vi "Update Count.vi"(8 "error in (no error)":errorcluster, 10 "Count":u64, 11 "Work Logic in":refnum<class "Work Logic.lvclass">) -> (0 "error out":errorcluster, 3 "Work Logic out":refnum<class "Work Logic.lvclass">)   [LabVIEW 2024, in "Chef State Logic.lvlib" / "Work Logic.lvclass"]
uses:
  Work Logic.lvclass
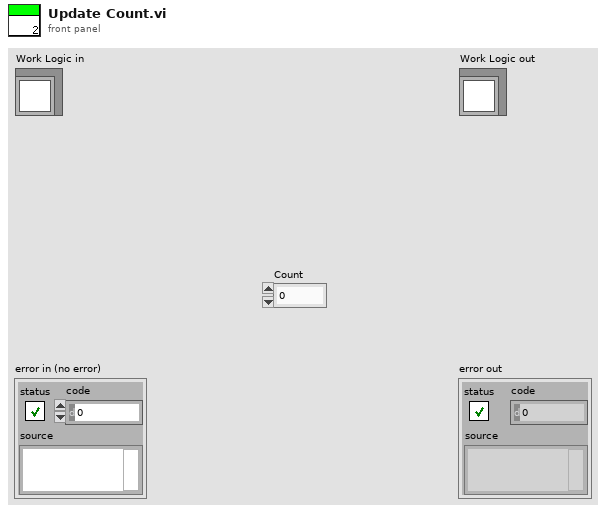
[diagram p1: front panel]
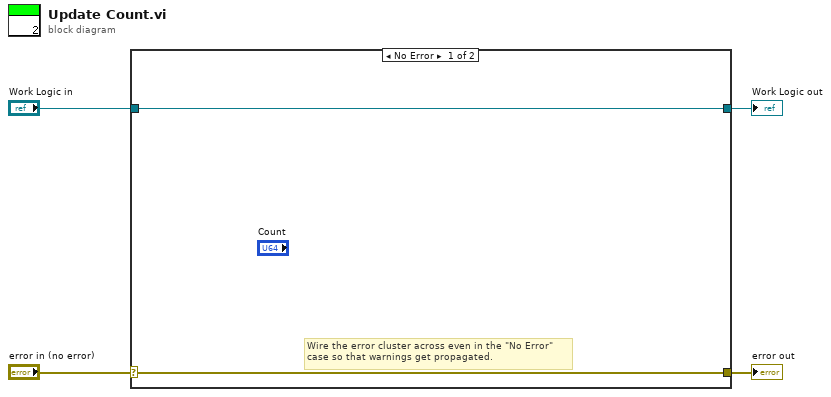
[diagram p0: block diagram]
diagram:
  n1 = case shown="No Error" "error in (no error)" {
    selector: "error in (no error)" -> [w5 w8]
    tunnel: [w5 w8] -> w3
    tunnel: [w6 w7] -> w1
    tunnel: "Work Logic in" -> [w6 w7]
    frame No Error {
      # "Wire the error cluster across even in the \"No Error\"\ncase so that warnings get propagated."
    }
    frame Error {
    }
  }
  "error out" <- w3
  "Work Logic out" <- w1
